vi "RSNRPZ Set Scope Measurements Offset Time.vi"(8 "error in (no error)":errorcluster, 9 "Offset Time (0.0 s)":dbl format="%^.3e", 10 "Channel (1)":i32=1, 11 "VISA session":refnum<visa-resource-name> caption="VISA resource name") -> (0 "error out":errorcluster, 3 "dup VISA session":refnum<visa-resource-name> caption="VISA resource name")   [LabVIEW 2010]
doc: "This VI defines offset time used to set the start point of analysing the current trace for the pulse parameters. The offset time could be used to start analysis from the second (or any other) pulse occurrence in the trace and not from the beginning of the trace.\n\nNote:\n1) This VI is only available for NRP-Z81.\n\nRemote-control command(s):\nSENSe:TRACe:MEAS:OFFS:TIME"
uses:
  rsnrpz_32.dll
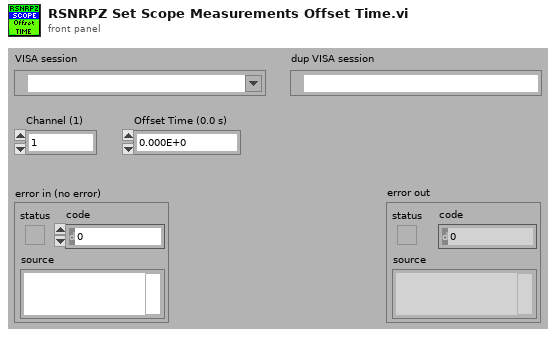
[diagram p1: front panel]
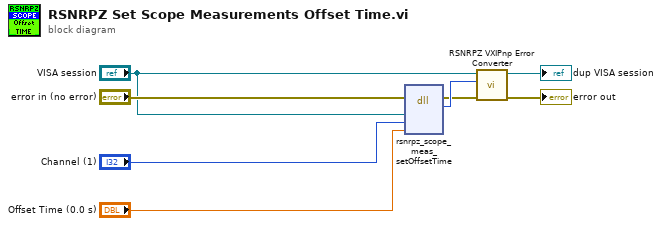
[diagram p0: block diagram]
diagram:
  n1 = dll-call lib="rsnrpz_32.dll" fn="rsnrpz_scope_meas_setOffsetTime"(error in="error in (no error)", "Instrument Handle"="VISA session", "Channel"="Channel (1)", "Offset Time"="Offset Time (0.0 s)") -> (error out=w5:errorcluster, "Status"=w8:i32)  [unwired: 5 in, 1 out]
  n2 = call <instrlib>:"RSNRPZ VXIPnp Error Converter.vi"("error in"=w5, "VXIPnp error code"=w8, "VISA session"="VISA session") -> ("error out"=→"error out":errorcluster, "dup VISA session"=→"dup VISA session":refnum<visa-resource-name>)  [unwired: 7 in]
